vi "nibbles2byte.vi"(2 "high nibble":u8, 3 "low nibble":u8) -> (7 "byte":u8)   [LabVIEW 2013]
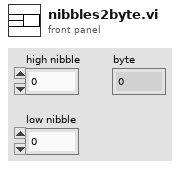
[diagram p1: front panel]
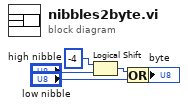
[diagram p0: block diagram]
diagram:
  n1 = Logical Shift(y=i16 -4, x="high nibble") -> (x << y=w3:u8)
  n2 = Or(x=w3, y="low nibble") -> (x .or. y?=→"byte":u8)
